vi "App Data.vi"() -> ()   [LabVIEW 2015]
panel:
  in  "device name":tag="myDAQ1"
  in  "Acq Time [ms]":dbl
  in  "Frequency [Hz]":dbl
  in  "Acquisition Loop Error":errorcluster
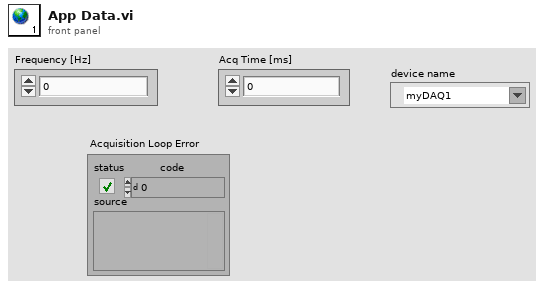
[diagram p1: front panel]
diagram:
